vi "Menu Selection (User).vi"(8 "error in (no error)":errorcluster, 9 "ItemPath":string, 10 "ItemTag":string, 11 "MCLB_Template in":refnum<class "MCLB_Template.lvclass">) -> (0 "error out":errorcluster, 3 "MCLB_Template out":refnum<class "MCLB_Template.lvclass">)   [LabVIEW 2021, in "MCLB_Template.lvclass"]
doc: "Menu Selection (User).vi"
uses:
  MCLB_Template.lvclass
  MouseSelect.ctl
  MCLB_Template.lvclass/MCLB_Template.ctl
panel:
  out "current time":timestamp
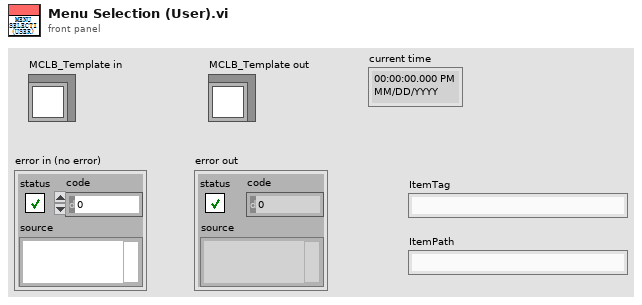
[diagram p1: front panel]
types:
  T1 = typedef "MCLB_Template.lvclass/MouseSelect.ctl" = cluster{"MouseDown Index":i32, "MouseUp Index":i32, "Mouse Move Index Array":i32[]}
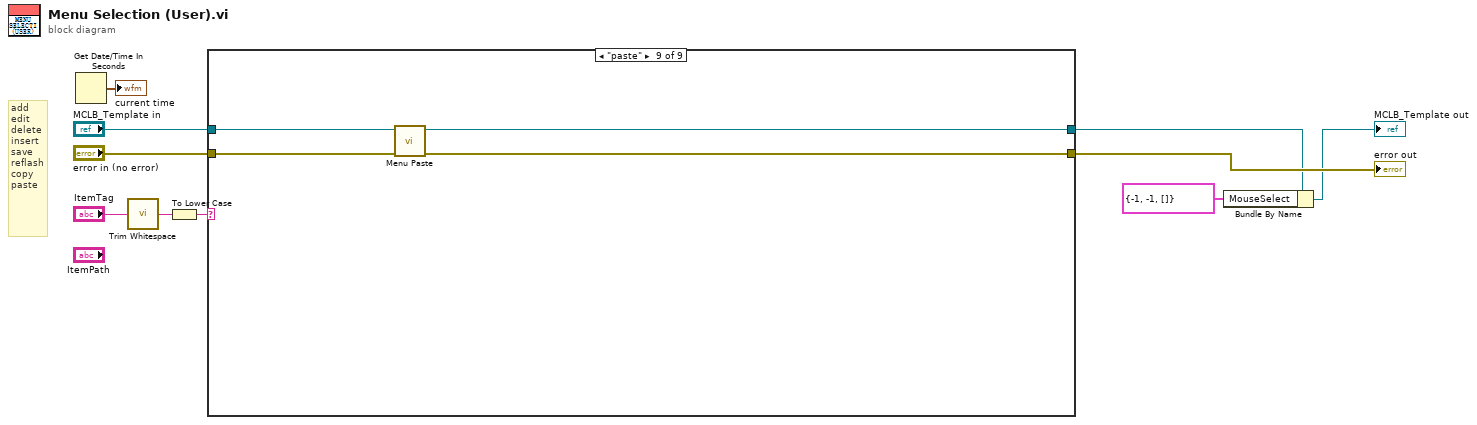
[diagram p0: block diagram]
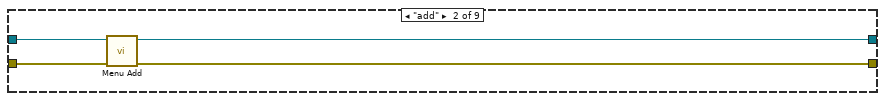
[diagram p3: hidden frame]
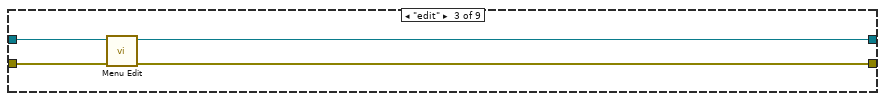
[diagram p4: hidden frame]
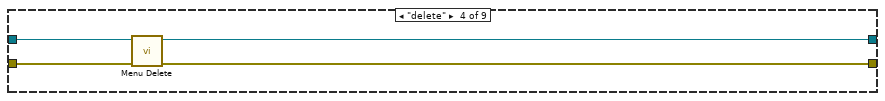
[diagram p5: hidden frame]
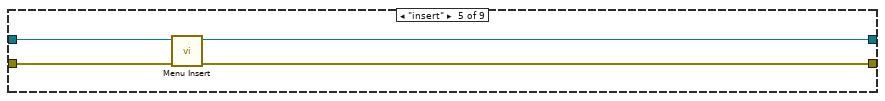
[diagram p6: hidden frame]
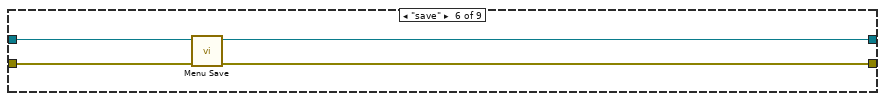
[diagram p7: hidden frame]
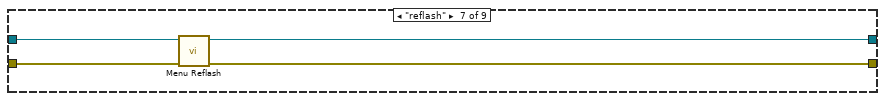
[diagram p8: hidden frame]
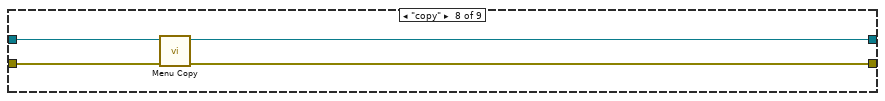
[diagram p9: hidden frame]
diagram:
  # "add\nedit\ndelete\ninsert\nsave\nreflash\ncopy\npaste"
  n1 = Get Date/Time In Seconds() -> (seconds since 1Jan1904=→"current time":timestamp)
  n2 = call <vilib>:"Trim Whitespace.vi"("string"="ItemTag") -> ("trimmed string"=w5:string)  [unwired: 1 in]
  n3 = To Lower Case(string=w5) -> (all lower case string=w6:string)
  n4 = case shown="\"paste\"" w6 {
    tunnel: "MCLB_Template in" -> [w12 w15 w19 w23 w27 w31 w35 w39 w43]
    tunnel: "error in (no error)" -> [w11 w13 w17 w21 w25 w29 w33 w37 w41]
    tunnel: [w12 w16 w20 w24 w28 w32 w36 w40 w44] -> w1
    tunnel: [w11 w14 w18 w22 w26 w30 w34 w38 w42] -> w7
    frame "False", Default {
    }
    frame "add" {
      n5 = call "Menu Add.vi"("error in (no error)"=w13, "MCLB_Template in"=w15) -> ("error out"=w14:errorcluster, "MCLB_Template out"=w16:refnum<class "MCLB_Template.lvclass">)  [unwired: 8 in]
    }
    frame "edit" {
      n6 = call "Menu Edit.vi"("error in (no error)"=w17, "MCLB_Template in"=w19) -> ("error out"=w18:errorcluster, "MCLB_Template out"=w20:refnum<class "MCLB_Template.lvclass">)  [unwired: 8 in]
    }
    frame "delete" {
      n7 = call "Menu Delete.vi"("error in (no error)"=w21, "MCLB_Template in"=w23) -> ("error out"=w22:errorcluster, "MCLB_Template out"=w24:refnum<class "MCLB_Template.lvclass">)  [unwired: 8 in]
    }
    frame "insert" {
      n8 = call "Menu Insert.vi"("error in (no error)"=w25, "MCLB_Template in"=w27) -> ("error out"=w26:errorcluster, "MCLB_Template out"=w28:refnum<class "MCLB_Template.lvclass">)  [unwired: 8 in]
    }
    frame "save" {
      n9 = call "Menu Save.vi"("error in (no error)"=w29, "MCLB_Template in"=w31) -> ("error out"=w30:errorcluster, "MCLB_Template out"=w32:refnum<class "MCLB_Template.lvclass">)  [unwired: 8 in]
    }
    frame "reflash" {
      n10 = call "Menu Reflash.vi"("error in (no error)"=w33, "MCLB_Template in"=w35) -> ("error out"=w34:errorcluster, "MCLB_Template out"=w36:refnum<class "MCLB_Template.lvclass">)  [unwired: 8 in]
    }
    frame "copy" {
      n11 = call "Menu Copy.vi"("error in (no error)"=w37, "MCLB_Template in"=w39) -> ("error out"=w38:errorcluster, "MCLB_Template out"=w40:refnum<class "MCLB_Template.lvclass">)  [unwired: 8 in]
    }
    frame "paste" {
      n12 = call "Menu Paste.vi"("error in (no error)"=w41, "MCLB_Template in"=w43) -> ("error out"=w42:errorcluster, "MCLB_Template out"=w44:refnum<class "MCLB_Template.lvclass">)  [unwired: 8 in]
    }
  }
  "error out" <- w7
  n13 = Bundle By Name(cluster=w1, "MouseSelect"=T1 {"MouseDown Index"=-1, "MouseUp Index"=-1, "Mouse Move Index Array"=[]}) -> (→"MCLB_Template out":refnum<class "MCLB_Template.lvclass">)
